vi "Finalize Channel.vi"(8 "error in":errorcluster, 10 "channel number":u8, 11 "board handle":u8) -> (0 "error out":errorcluster, 2 "channel number out":u8, 3 "board handle out":u8)   [LabVIEW 2020, in "AIM ARINC 429 Hardware API.lvlib"]
uses:
  AIM ARINC 429 Hardware API.lvlib
  <instrlib>/AIM GmbH/_ARINC-429/AIM429LV.lvlib
  Channel Action.ctl
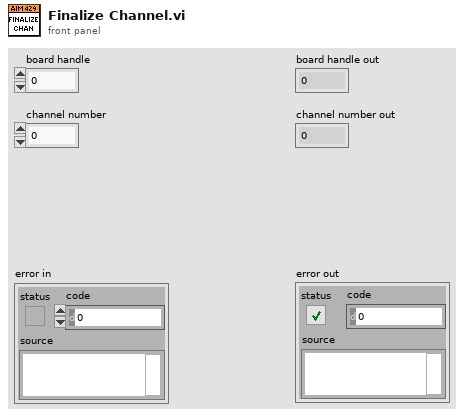
[diagram p1: front panel]
types:
  T1 = typedef "AIM ARINC 429 Hardware API.lvlib/Channel Action.ctl" = enum16{"Get Info", "Initialize", "Start", "Clear"}
  T2 = typedef "AIM ARINC 429 Hardware API.lvlib/Channel Status.ctl" = enum16{"Uninitialized", "Idle", "Active"}
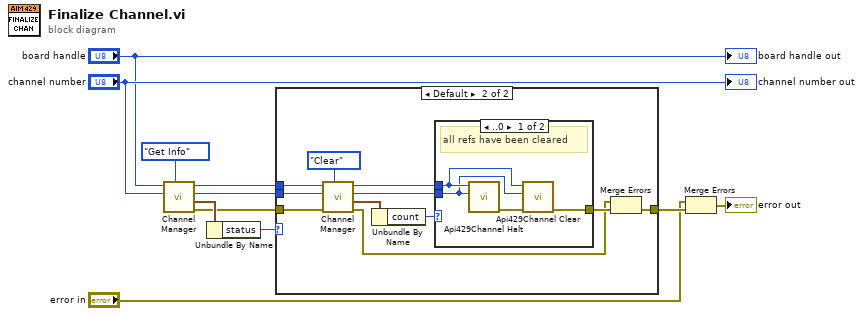
[diagram p0: block diagram]
diagram:
  n1 = call "Channel Manager.vi"("action"=Channel_Action."Get Info", "channel number"="channel number", "board handle"="board handle") -> ("error out"=w8:errorcluster, "channel info"=w10:cluster{"count":u32, "status":T2}, "channel number out"=w6:u8, "board handle out"=w7:u8)  [unwired: 5 in]
  n2 = Unbundle By Name(w10) -> ("status"=w9:T2)
  n3 = case shown="Default" w9 {
    tunnel: w8 -> [w12 w23]
    tunnel: w7 -> [_ w22]
    tunnel: w6 -> [_ w21]
    tunnel: [w12 w13] -> w5
    frame "Uninitialized" {
      # "no need to stop an uninitialized channel"
    }
    frame Default {
      n4 = call "Channel Manager.vi"("action"=Channel_Action."Clear", "error in"=w23, "channel number"=w21, "board handle"=w22) -> ("error out"=w14:errorcluster, "channel info"=w19:cluster{"count":u32, "status":T2}, "channel number out"=w16:u8, "board handle out"=w17:u8)  [unwired: 4 in]
      n5 = Unbundle By Name(w19) -> ("count"=w18:u32)
      n6 = case shown="..0" w18 {
        tunnel: w17 -> [w26 _]
        tunnel: w16 -> [w25 _]
        tunnel: [w24 _] -> w15
        frame ..0 {
          # "all refs have been cleared"
          n7 = call <instrlib>:"Api429Channel Halt.vi"("channel_id"=w25, "board_handle"=w26) -> ("error out"=w27:errorcluster)  [unwired: 9 in]
          n8 = call <instrlib>:"Api429Channel Clear.vi"("error in (no error)"=w27, "channel_id"=w25, "board_handle"=w26) -> ("error out"=w24:errorcluster)  [unwired: 8 in]
        }
        frame Default {
          # "something is still using the channel"
        }
      }
      n9 = Merge Errors(w14, w15) -> (w13:errorcluster)
    }
  }
  n10 = Merge Errors("error in", w5) -> (→"error out":errorcluster)
  "board handle out" <- "board handle"
  "channel number out" <- "channel number"
